vi "path.set.vi"(8 "error in (no error)":errorcluster, 10 "path":string, 11 "source in":refnum<class "source.lvclass">) -> (0 "error out":errorcluster, 3 "source out":refnum<class "source.lvclass">)   [LabVIEW 2020, in "datasources.lvlib" / "source.lvclass"]
uses:
  source.lvclass
  source.lvclass/source.ctl
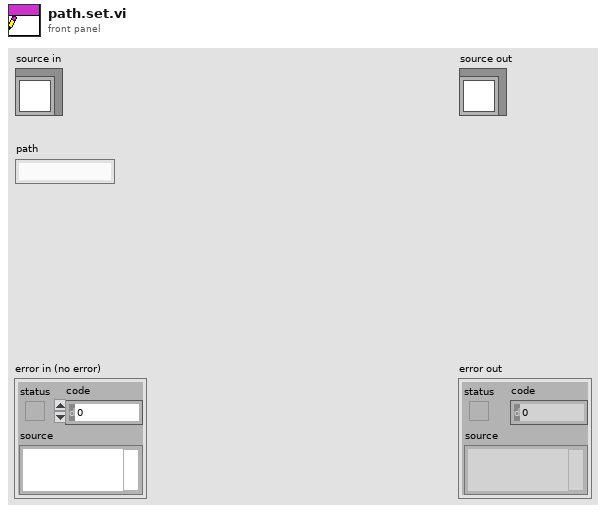
[diagram p1: front panel]
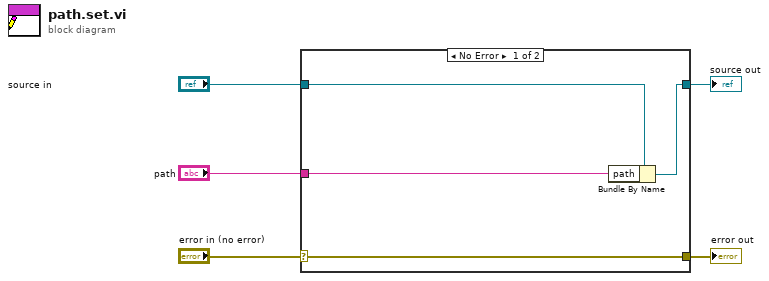
[diagram p0: block diagram]
diagram:
  n1 = case shown="No Error" "error in (no error)" {
    selector: "error in (no error)" -> [w9 w10]
    tunnel: [w9 w10] -> w4
    tunnel: [w7 w11] -> w2
    tunnel: "source in" -> [w8 w11]
    tunnel: "path" -> [w6 _]
    frame No Error {
      n2 = Bundle By Name(cluster=w8, "path"=w6) -> (w7:refnum<class "source.lvclass">)
    }
    frame Error {
    }
  }
  "error out" <- w4
  "source out" <- w2
